vi "LVClass_Camera Read synchronisation mode.vi"(8 "error in (no error)":errorcluster, 11 "Camera in":refnum<class "Camera.lvclass">) -> (0 "error out":errorcluster, 2 "synchronisation_mode":enum16{"synchronous", "asynchronous"}(ring), 3 "Camera out":refnum<class "Camera.lvclass">)   [LabVIEW 2020, in "Camera.lvclass"]
doc: "Get camera acquisition status\n\n<B>CameraIn</B> : Camera object.\n<B>CameraOut</B> : Camera object.\n<B>acquisition Mode</B> : acquisition modfe value (Last image, New image)"
uses:
  Camera.lvclass
  Camera.lvclass/Camera.ctl
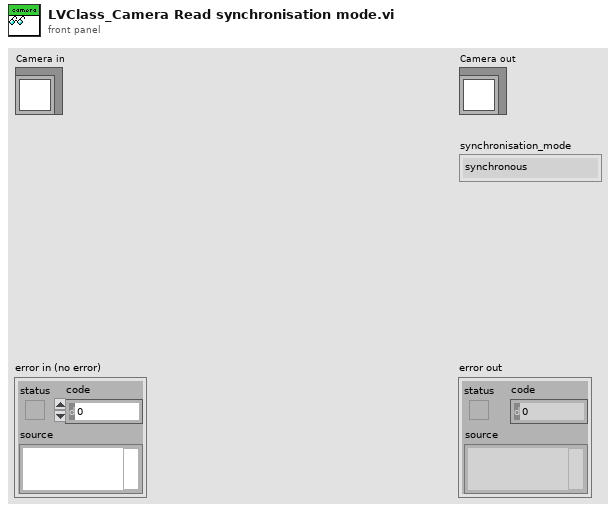
[diagram p1: front panel]
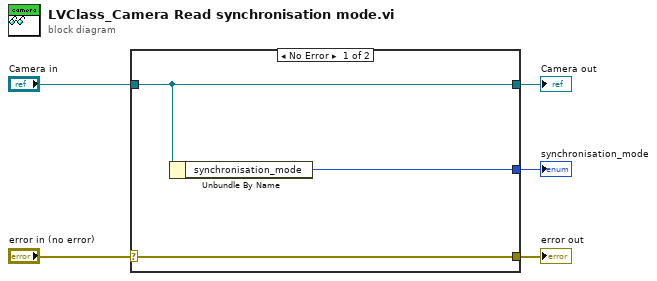
[diagram p0: block diagram]
diagram:
  n1 = case shown="No Error" "error in (no error)" {
    selector: "error in (no error)" -> [w8 w9]
    tunnel: [w8 w9] -> w4
    tunnel: [w7 w10] -> w2
    tunnel: "Camera in" -> [w7 w10]
    tunnel: [w6 _] -> w1
    frame No Error {
      n2 = Unbundle By Name(w7) -> ("synchronisation_mode"=w6:enum16{"synchronous", "asynchronous"})
    }
    frame Error {
    }
  }
  "error out" <- w4
  "Camera out" <- w2
  "synchronisation_mode" <- w1
